vi "ShutDown.vi"(8 "error in (no error)":errorcluster, 11 "TCP_ServerWithGUI in":refnum<class "TCP_ServerWithGUI.lvclass">) -> (0 "error out":errorcluster, 3 "TCP_ServerWithGUI out":refnum<class "TCP_ServerWithGUI.lvclass">)   [LabVIEW 2023, in "TCP_serverGUI.lvlib" / "TCP_ServerWithGUI.lvclass"]
uses:
  TCP_ServerWithGUI.lvclass
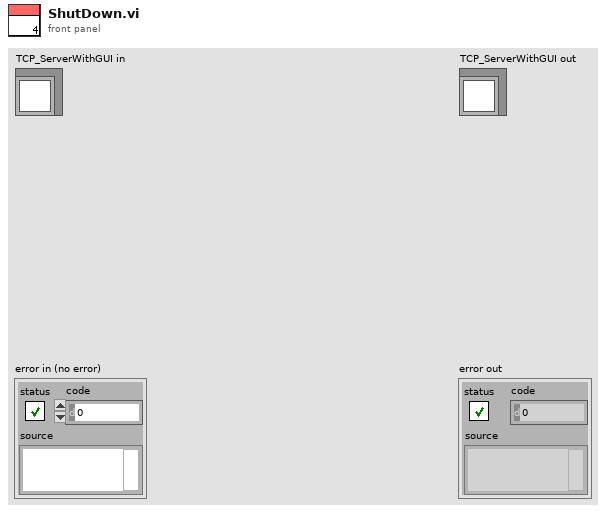
[diagram p1: front panel]
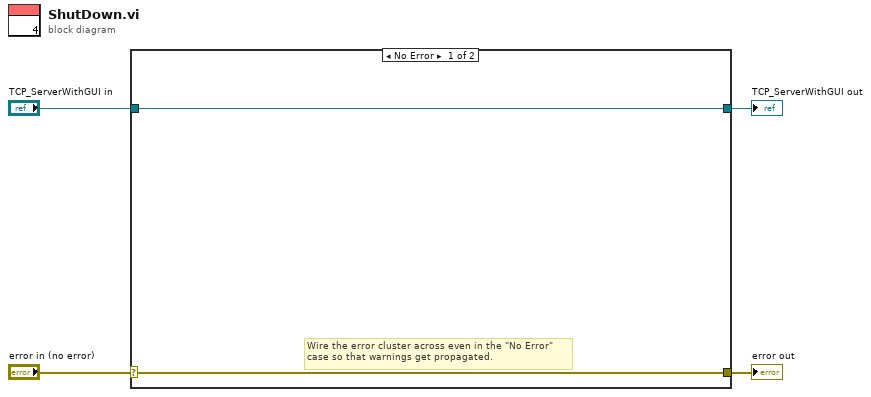
[diagram p0: block diagram]
diagram:
  n1 = case shown="No Error" "error in (no error)" {
    selector: "error in (no error)" -> [w5 w8]
    tunnel: [w5 w8] -> w3
    tunnel: [w6 w7] -> w1
    tunnel: "TCP_ServerWithGUI in" -> [w6 w7]
    frame No Error {
      # "Wire the error cluster across even in the \"No Error\"\ncase so that warnings get propagated."
    }
    frame Error {
    }
  }
  "error out" <- w3
  "TCP_ServerWithGUI out" <- w1
